vi "Configure Window Dialog.vi"(5 "New":bool, 6 "degrees of one u16":dbl, 7 "Window to be edited":i32, 8 "error in (no error)":errorcluster, 9 "Max engine angle":dbl min=0.0 format="%#_f", 10 "windows in":T1[](array[typedef]), 11 "Item Ref in":T2 format="%.0x") -> (0 "error out":errorcluster, 2 "windows out":T1[](array[typedef]), 3 "Item Ref out":T2 format="%.0x")   [LabVIEW 2017, in "Engine Simulation Toolkit System Explorer.lvlib"]
uses:
  Engine Simulation Toolkit System Explorer.lvlib
  Event Timing Window.ctl
  <vilib>/NI Veristand/Custom Device API/Custom Device Item Ref.ctl
  <vilib>/NI Veristand/Custom Device API/Custom Device API.lvlib
panel:
  in  "Reference angle (degrees)":dbl
  in  "Cancel":bool
  in  "OK":bool
  in  "Maximum angle (degrees)":dbl
  in  "Minimum angle (degrees)":dbl
  in  "Name":string
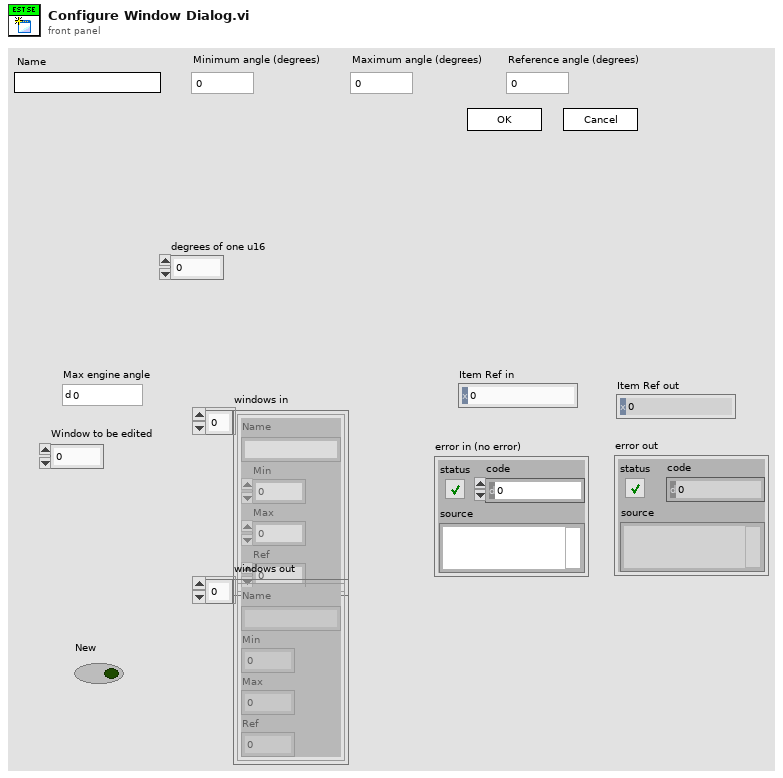
[diagram p1: front panel]
types:
  T1 = typedef "Engine Simulation Toolkit System Explorer.lvlib/Event Timing Window.ctl" = cluster{"Name":string, "Min":dbl, "Max":dbl, "Ref":dbl}
  T2 = typedef "Custom Device API.lvlib/Custom Device Item Ref.ctl" = u64
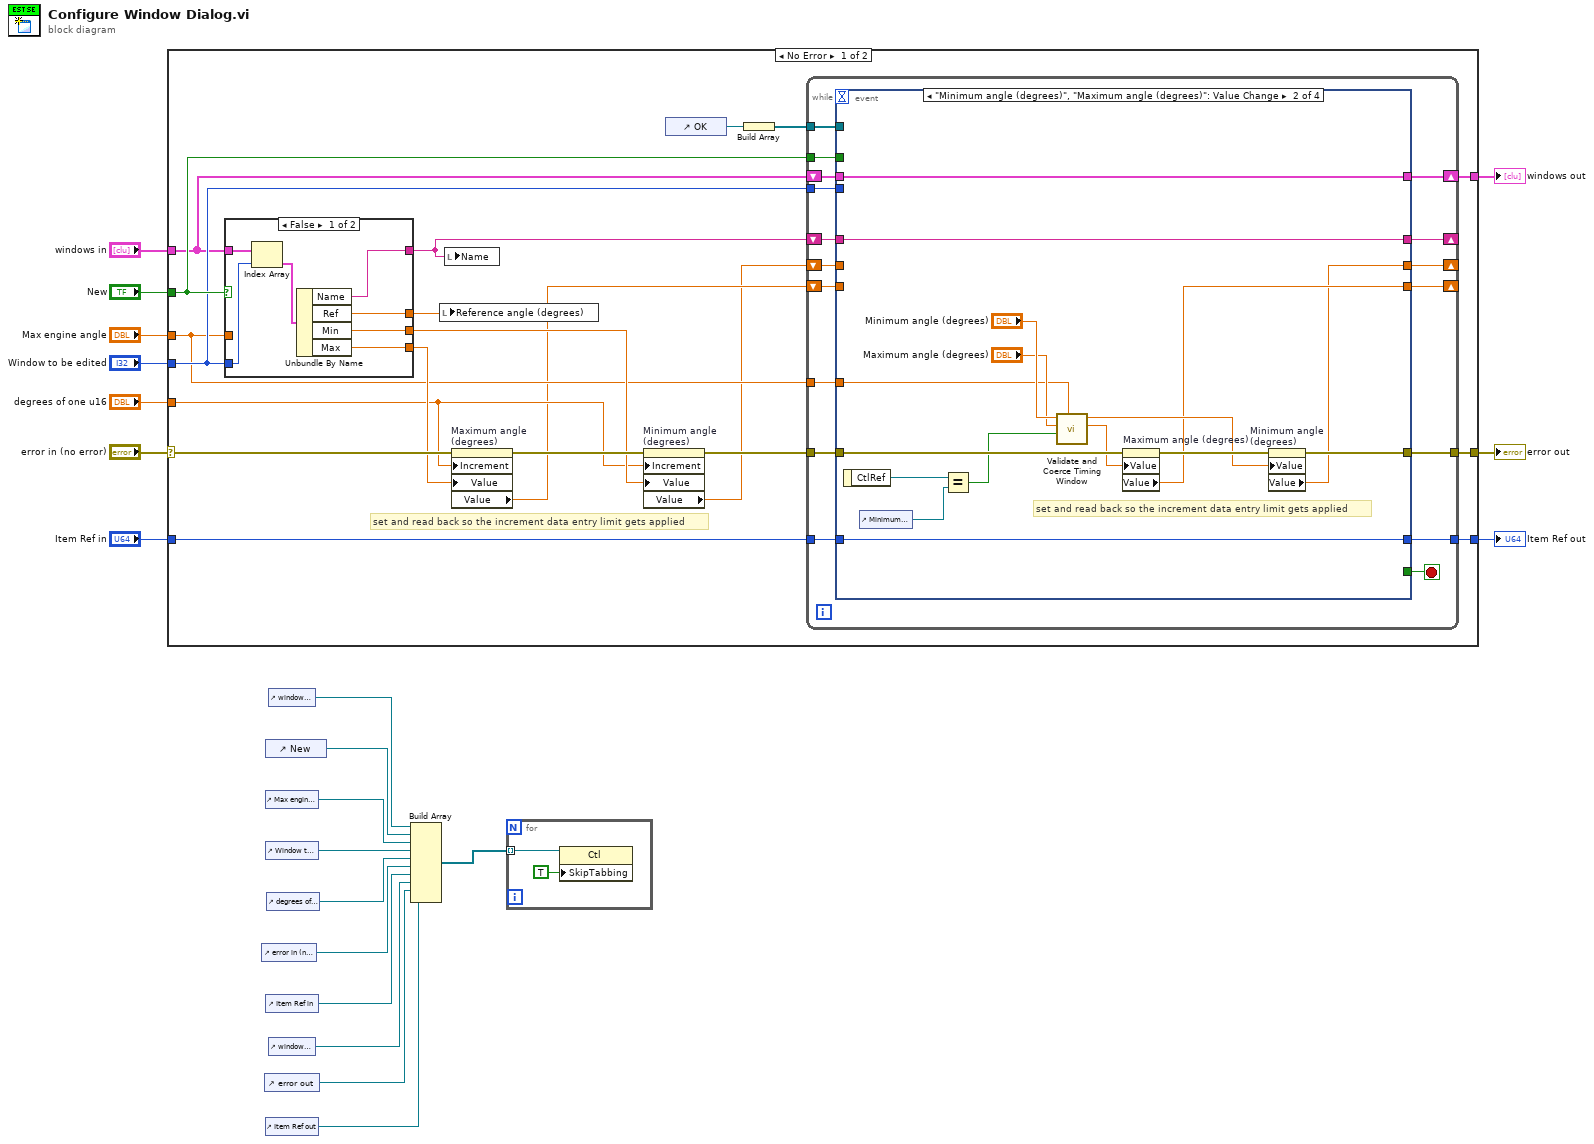
[diagram p0: block diagram]
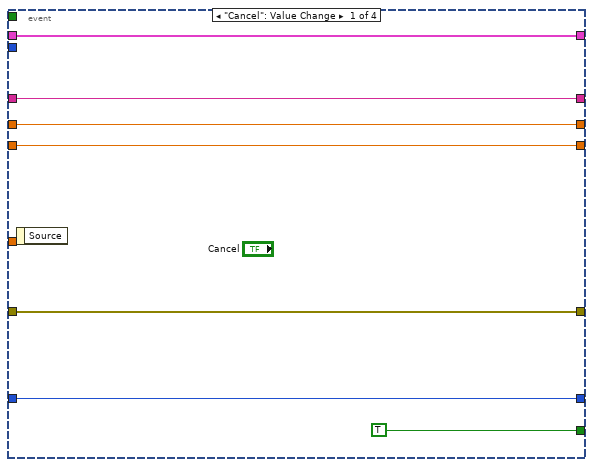
[diagram p2: hidden frame]
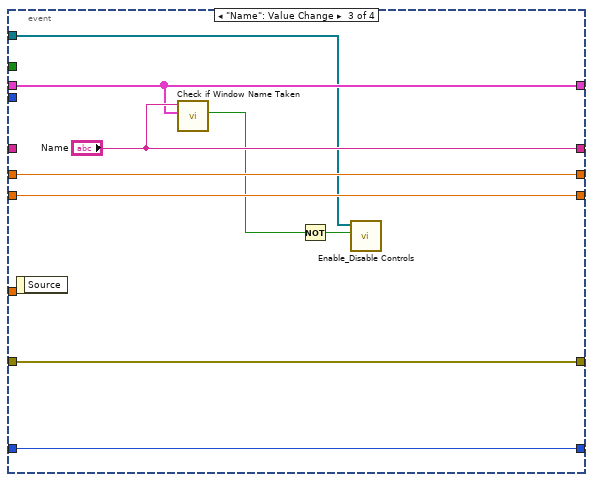
[diagram p3: hidden frame]
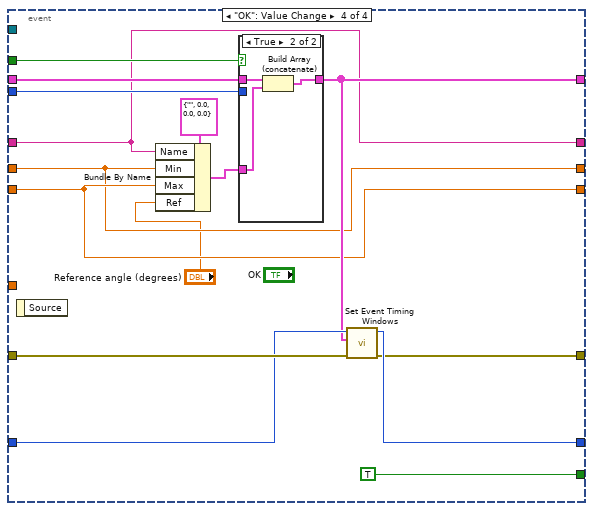
[diagram p4: hidden frame]
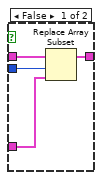
[diagram p5: hidden frame]
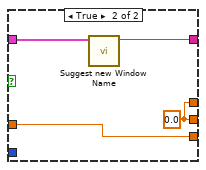
[diagram p6: hidden frame]
diagram:
  n1 = case shown="No Error" "error in (no error)" {
    selector: "error in (no error)" -> [w41 w126]
    tunnel: "New" -> [w37 _]
    tunnel: "windows in" -> [w35 w125]
    tunnel: "Max engine angle" -> [w25 _]
    tunnel: "Window to be edited" -> [w36 _]
    tunnel: "degrees of one u16" -> [w26 _]
    tunnel: [w39 w126] -> w15
    tunnel: [w34 w125] -> w14
    tunnel: "Item Ref in" -> [w33 w124]
    tunnel: [w32 w124] -> w12
    frame No Error {
      # "set and read back so the increment data entry limit gets applied"
      n2 = case shown="False" w37 {
        tunnel: w35 -> [w116 w123]
        tunnel: w25 -> [_ w121]
        tunnel: [w118 w120] -> w30
        tunnel: [w117 w121] -> w27
        tunnel: w36 -> [w115 _]
        tunnel: [w119 w122] -> w31
        tunnel: [w113 w120] -> w22
        frame False {
          n3 = Index Array(array=w116, index=w115) -> (element=w114:T1)
          n4 = Unbundle By Name(w114) -> ("Name"=w119:string, "Ref"=w113:dbl, "Min"=w118:dbl, "Max"=w117:dbl)
        }
        frame True {
          w120 = 0.0 ("Min")
          n5 = call "Suggest new Window Name.vi"("windows in"=w123) -> ("suggested name"=w122:string)  [unwired: 10 in]
        }
      }
      n6 = local write "Reference angle (degrees)"(w22) -> ()
      n7 = local write "Name"(w31) -> ()
      n8 = property on="Maximum angle (degrees)" class="DigNum (strict)"(error in=w41, "Increment"=w26, "Value"=w27) -> (error out=w40:errorcluster, "Value"=w24:dbl)  [unwired: 1 in, 1 out]
      n9 = property on="Minimum angle (degrees)" class="DigNum (strict)"(error in=w40, "Increment"=w26, "Value"=w30) -> (error out=w38:errorcluster, "Value"=w23:dbl)  [unwired: 1 in, 1 out]
      n10 = control-ref of="OK"() -> (w29:refnum<vi>)
      n11 = Build Array(w29) -> (w28:refnum<vi>[])
      n12 = while {
        tunnel: [w44] -> w39
        tunnel: w38 -> [w58]
        tunnel: w37 -> [w57]
        tunnel: w36 -> [w56]
        tunnel: w33 -> [w53]
        tunnel: [w52] -> w32
        shift-right: [w50] -> _
        shift-left: w31 -> [w49]
        shift-right: [w48] -> _
        shift-left: w23 -> [w47]
        shift-right: [w46] -> _
        shift-left: w24 -> [w45]
        tunnel: w28 -> [w43]
        tunnel: w25 -> [w42]
        shift-right: [w54] -> w34
        shift-left: w35 -> [w55]
        stop <- w51 stop-if-true
        n13 = event shown="[1] \"Minimum angle (degrees)\", \"Maximum angle (degrees)\": Value Change" {
          selector: _ -> [_ _ _ _]
          dyn-events: _ -> [_ _ _ _]
          timeout: _ -> [_ _ _ _]
          tunnel: [w65 w77 w85 w97] -> w44
          tunnel: w58 -> [w65 w76 w85 w100]
          tunnel: w57 -> [_ _ _ w105]
          tunnel: w56 -> [_ _ _ w103]
          tunnel: w55 -> [w64 w80 w86 w104]
          tunnel: [w64 w80 w86 w96] -> w54
          tunnel: w53 -> [w63 w81 w90 w99]
          tunnel: [w63 w81 w90 w98] -> w52
          tunnel: [TRUE _ _ TRUE] -> w51
          tunnel: w47 -> [w61 _ w89 w92]
          tunnel: w45 -> [w60 _ w88 w93]
          tunnel: [w59 w79 "Name" w94] -> w50
          tunnel: w49 -> [w59 w79 _ w94]
          tunnel: [w61 w66 w89 w92] -> w48
          tunnel: [w60 w67 w88 w93] -> w46
          tunnel: w43 -> [_ _ w84 _]
          tunnel: w42 -> [_ w70 _ _]
          event "Cancel": Value Change {
            n14 = event-data() -> ()  [unwired: 1 in, 1 out]
          }
          event "Minimum angle (degrees)", "Maximum angle (degrees)": Value Change {
            # "set and read back so the increment data entry limit gets applied"
            n15 = event-data() -> ("CtlRef"=w75:refnum<vi>)  [unwired: 1 in]
            n16 = control-ref of="Minimum angle (degrees)"() -> (w74:refnum<vi>)
            n17 = Equal?(x=w75, y=w74) -> (x = y?=w73:bool)
            n18 = call "Validate and Coerce Timing Window.vi"("Max engine angle"=w70, "Min changed last"=w73, "Max"="Maximum angle (degrees)", "Min"="Minimum angle (degrees)") -> ("Coerced maximum"=w68:dbl, "Coerced minimum"=w69:dbl)  [unwired: 6 in]
            n19 = property on="Maximum angle (degrees)" class="DigNum (strict)"(error in=w76, "Value"=w68) -> (error out=w78:errorcluster, "Value"=w67:dbl)  [unwired: 1 in, 1 out]
            n20 = property on="Minimum angle (degrees)" class="DigNum (strict)"(error in=w78, "Value"=w69) -> (error out=w77:errorcluster, "Value"=w66:dbl)  [unwired: 1 in, 1 out]
          }
          event "Name": Value Change {
            n21 = event-data() -> ()  [unwired: 1 in, 1 out]
            n22 = call "Check if Window Name Taken.vi"("windows in"=w86, "name"="Name") -> ("taken"=w82:bool)  [unwired: 9 in]
            n23 = Not(x=w82) -> (.not. x?=w83:bool)
            n24 = call "Enable_Disable Controls.vi"("Enable?"=w83, "Controls"=w84) -> ()  [unwired: 10 in]
          }
          event "OK": Value Change {
            n25 = event-data() -> ()  [unwired: 1 in, 1 out]
            n26 = Bundle By Name(cluster=T1 {"Name"="", "Min"=0.0, "Max"=0.0, "Ref"=0.0} ("new element/subarray"), "Name"=w94, "Min"=w92, "Max"=w93, "Ref"="Reference angle (degrees)") -> (w101:T1)
            n27 = case shown="True" w105 {
              tunnel: w104 -> [w109 w112]
              tunnel: w103 -> [w108 _]
              tunnel: [w107 w110] -> w96
              tunnel: w101 -> [w106 w111]
              frame False {
                n28 = Replace Array Subset(array=w109, new element=w106, index=w108) -> (w107:T1[])
              }
              frame True {
                n29 = Build Array (concatenate)(w112, w111) -> (w110:T1[])
              }
            }
            n30 = call "Set Event Timing Windows.vi"("error in (no error)"=w100, "Windows"=w96, "Item Ref in"=w99) -> ("error out"=w97:errorcluster, "Item Ref out"=w98:T2)  [unwired: 7 in]
          }
        }
      }
    }
    frame Error {
    }
  }
  "error out" <- w15
  "Item Ref out" <- w12
  "windows out" <- w14
  n31 = control-ref of="error in (no error)"() -> (w6:refnum<vi>)
  n32 = control-ref of="error out"() -> (w2:refnum<vi>)
  n33 = control-ref of="New"() -> (w10:refnum<vi>)
  n34 = control-ref of="Max engine angle"() -> (w9:refnum<vi>)
  n35 = control-ref of="Window to be edited"() -> (w8:refnum<vi>)
  n36 = control-ref of="Item Ref in"() -> (w5:refnum<vi>)
  n37 = control-ref of="Item Ref out"() -> (w1:refnum<vi>)
  n38 = control-ref of="degrees of one u16"() -> (w7:refnum<vi>)
  n39 = control-ref of="windows in"() -> (w11:refnum<vi>)
  n40 = control-ref of="windows out"() -> (w3:refnum<vi>)
  n41 = Build Array(w11, w10, w9, w8, w7, w6, w5, w3, w2, w1) -> (w4:refnum<vi>[])
  n42 = for {
    tunnel: w4 -> [w128] mode=indexing
    n43 = property class="Ctl"(reference=w128, "SkipTabbing"=TRUE ("Skip When Tabbing")) -> ()  [unwired: 1 in, 2 out]
  }
